vi "Init if Unset.vi"(4 "Value Tree in":refnum<class "Value Tree.lvclass">, 5 "Type (Object)":T1=enum."Object") -> (7 "Value Tree out":refnum<class "Value Tree.lvclass">)   [LabVIEW 2020, in "HTTP Server.lvlib" / "Value Tree.lvclass"]
uses:
  Value Tree.lvclass
  Value Tree.lvclass/Value Tree.ctl
  Local Type.ctl
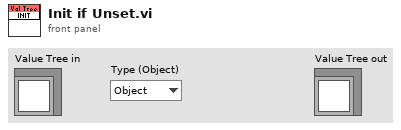
[diagram p1: front panel]
types:
  T1 = typedef "HTTP Server.lvlib/Value Tree.lvclass/Local Type.ctl" = enum16{"Scalar", "Object", "Array"}
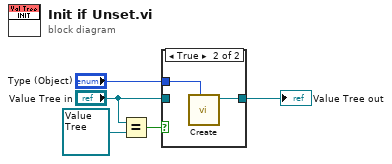
[diagram p0: block diagram]
diagram:
  n1 = Equal?(x="Value Tree in", y=refnum<class "Value Tree.lvclass"> refnum) -> (x = y?=w4:bool)
  n2 = case shown="True" w4 {
    tunnel: "Value Tree in" -> [w6 _]
    tunnel: "Type (Object)" -> [_ w7]
    tunnel: [w6 w8] -> w1
    frame False {
    }
    frame True {
      n3 = call "Create.vi"("Root Type (Scalar)"=w7) -> ("Value Tree out"=w8:refnum<class "Value Tree.lvclass">)  [unwired: 10 in]
    }
  }
  "Value Tree out" <- w1
